vi "Check-Mapping-storage.vi"(7 "Save?":bool, 8 "error in":errorcluster, 9 "Temp. params. ref.":refnum<data-value>, 10 "Analysis params. ref.":refnum<data-value>, 11 "Mapping params. ref.":refnum<data-value>) -> (0 "error IO":errorcluster, 3 "Passed?":bool)   [LabVIEW 2013, in "CameraVision.lvlib" / "CV-Storage.lvclass"]
uses:
  CV-Storage.lvclass
  Mapping/CV-Mapping.lvclass
  Analysis/CV-Analysis.lvclass
  Temperature/CV-Temperature.lvclass
  Analysis/CV-Analysis.lvclass/CV-Analysis.ctl
  Mapping/CV-Mapping.lvclass/CV-Mapping.ctl
  Mapping/Read Enable mapping.vi
  Analysis/Read Image characteristics.vi
  Analysis/Read Melt-pool characteristics.vi
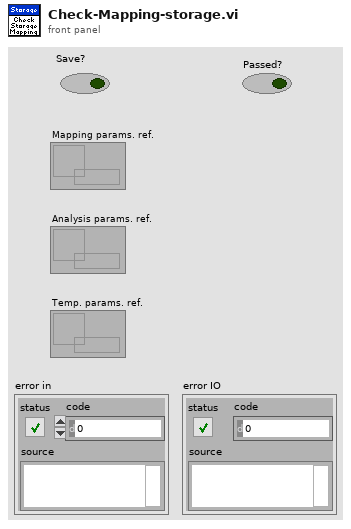
[diagram p1: front panel]
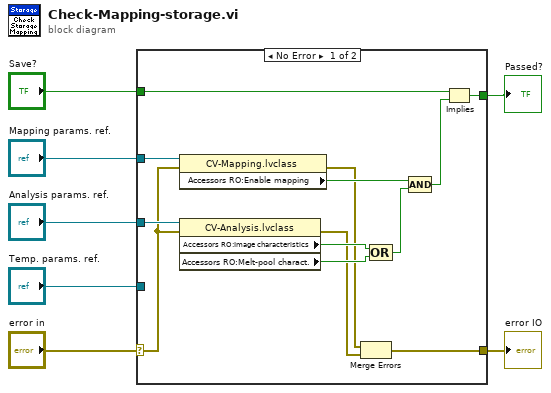
[diagram p0: block diagram]
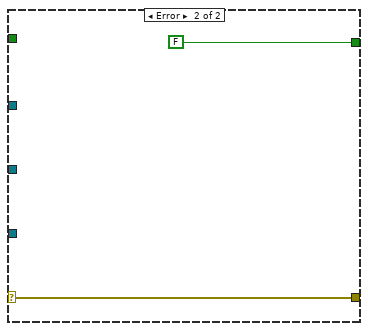
[diagram p2: hidden frame]
diagram:
  n1 = case shown="No Error" "error in" {
    selector: "error in" -> [w11 w21]
    tunnel: "Temp. params. ref." -> [_ _]
    tunnel: [w8 w21] -> w6
    tunnel: [w19 FALSE] -> w7
    tunnel: "Save?" -> [w18 _]
    tunnel: "Analysis params. ref." -> [w14 _]
    tunnel: "Mapping params. ref." -> [w16 _]
    frame No Error {
      n2 = property class="CV-Mapping.lvclass"(reference=w16, error in=w11) -> (error out=w10:errorcluster, "Accessors RO:Enable mapping"=w15:bool)  [unwired: 1 out]
      n3 = property class="CV-Analysis.lvclass"(reference=w14, error in=w11) -> (error out=w9:errorcluster, "Accessors RO:Image characteristics"=w13:bool, "Accessors RO:Melt-pool charact."=w12:bool)  [unwired: 1 out]
      n4 = Merge Errors(w10, w9) -> (w8:errorcluster)
      n5 = Compound Arithmetic op=OR(w13, w12) -> (w17:bool)
      n6 = Compound Arithmetic op=AND(w15, w17) -> (w20:bool)
      n7 = Implies(1:w20, 2:w18) -> (0:w19:bool)
    }
    frame Error {
    }
  }
  "Passed?" <- w7
  "error IO" <- w6
